vi "Set Channel PWM.vi"(8 "error in (no error)":errorcluster, 9 "Channel":u8, 10 "Duty Cycle 50%)":dbl=50.0, 11 "PWM in":refnum<class "LINX-PCA9865 PWM.lvclass">) -> (0 "error out":errorcluster, 3 "PWM out":refnum<class "LINX-PCA9865 PWM.lvclass">)   [LabVIEW 2019, in "LINX-PCA9865 PWM.lvclass"]
uses:
  LINX-PCA9865 PWM.lvclass
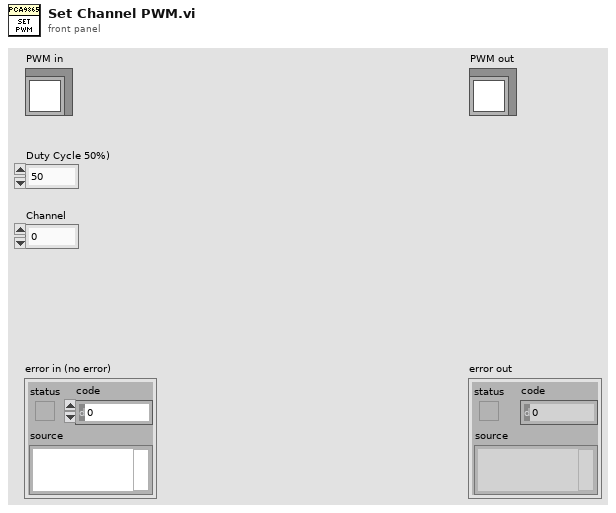
[diagram p1: front panel]
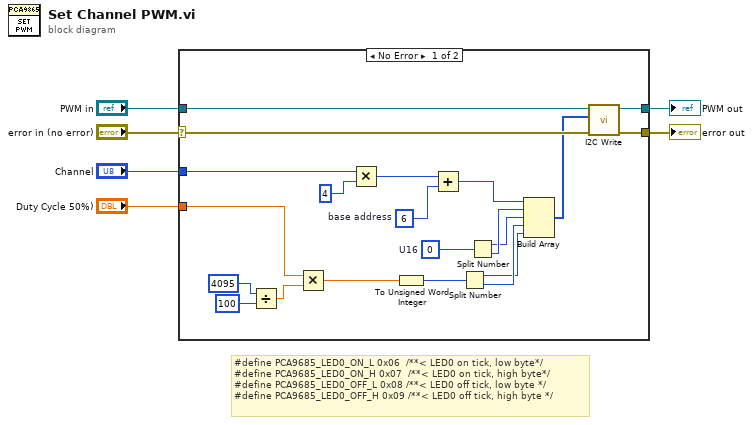
[diagram p0: block diagram]
diagram:
  # "#define PCA9685_LED0_ON_L 0x06  /**< LED0 on tick, low byte*/\n#define PCA9685_LED0_ON_H 0x07  /**< LED0 on tick, high byte*/\n#define PCA9685_LED0_OFF_L 0x08 /**< LED0 off tick, low byte */\n#define PCA9685_LED0_OFF_H 0x09 /**< LED0 off tick, high byte */"
  n1 = case shown="No Error" "error in (no error)" {
    selector: "error in (no error)" -> [w26 w29]
    tunnel: [w25 w29] -> w5
    tunnel: [w24 w28] -> w3
    tunnel: "PWM in" -> [w27 w28]
    tunnel: "Channel" -> [w23 _]
    tunnel: "Duty Cycle 50%)" -> [w14 _]
    frame No Error {
      w13 = u16 0  # U16
      w20 = u8 6  # base address
      n2 = Divide(x=4095, y=100) -> (x/y=w15:dbl)
      n3 = Multiply(x=w14, y=w15) -> (x*y=w10:dbl)
      n4 = Multiply(x=w23, y=u8 4) -> (x*y=w21:u8)
      n5 = To Unsigned Word Integer(number=w10) -> (unsigned 16bit integer=w9:u16)
      n6 = Add(x=w21, y=w20) -> (x+y=w19:u8)
      n7 = Split Number(x=w9) -> (hi(x)=w7:u8, lo(x)=w8:u8)
      n8 = Split Number(x=w13) -> (hi(x)=w11:u8, lo(x)=w12:u8)
      n9 = Build Array(w19, w12, w11, w8, w7) -> (w18:u8[])
      n10 = call "I2C Write.vi"("error in (no error)"=w26, "Bytes to Write"=w18, "LINX-PCA9865 PWM in"=w27) -> ("error out"=w25:errorcluster, "LINX-PCA9865 PWM out"=w24:refnum<class "LINX-PCA9865 PWM.lvclass">)  [unwired: 7 in]
    }
    frame Error {
    }
  }
  "error out" <- w5
  "PWM out" <- w3
